vi "Supply_ComplianceCheck.vi"(8 "error in (no error)":errorcluster, 11 "KE2657A in":refnum<class "KE2657A.lvclass">) -> (0 "error out":errorcluster, 1 "Status string":string, 2 "Compliance exceeded?":bool, 3 "KE2657A out":refnum<class "KE2657A.lvclass">)   [LabVIEW 2018]
uses:
  KE2657A.lvclass
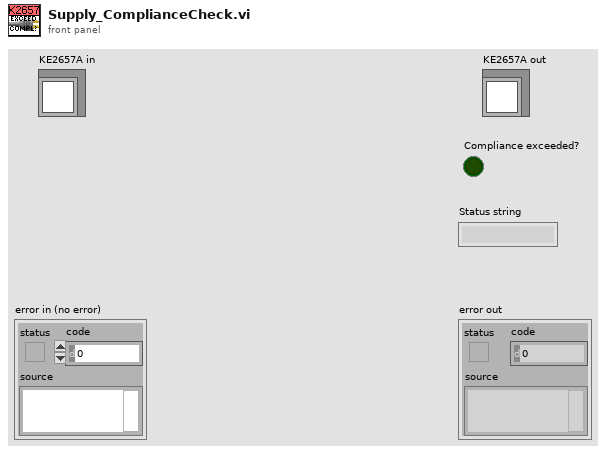
[diagram p1: front panel]
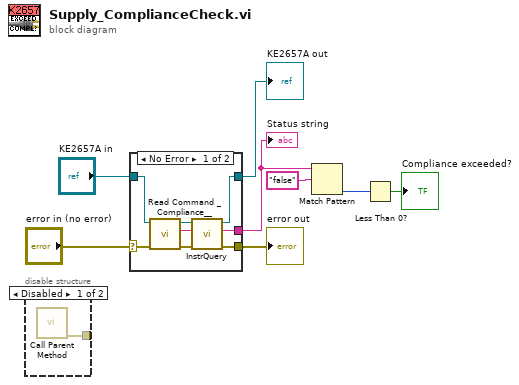
[diagram p0: block diagram]
diagram:
  n1 = disable-structure shown="Disabled" {
    disable-tunnel: [w9 _] -> _
    frame Disabled {
      n2 = call-parent "Call Parent Method"() -> ("error out"=w9:errorcluster)  [unwired: 8 in, 3 out]
    }
    frame Enabled {
    }
  }
  n3 = case shown="No Error" "error in (no error)" {
    selector: "error in (no error)" -> [w10 w18]
    tunnel: [w17 w18] -> w5
    tunnel: [w16 w19] -> w6
    tunnel: "KE2657A in" -> [w12 w19]
    tunnel: [w11 _] -> w4
    frame No Error {
      n4 = call-dynamic "Read Command _Compliance__.vi"("error in (no error)"=w10, "SupplyControl in"=w12) -> ("error out"=w15:errorcluster, "Command \"Compliance?\""=w14:string, "SupplyControl out"=w13:refnum<class "KE2657A.lvclass">)  [unwired: 7 in]
      n5 = call-dynamic "InstrQuery.vi"("error in (no error)"=w15, "Command string"=w14, "InstControl in"=w13) -> ("error out"=w17:errorcluster, "Instrument response"=w11:string, "InstControl out"=w16:refnum<class "KE2657A.lvclass">)  [unwired: 6 in]
    }
    frame Error {
    }
  }
  "KE2657A out" <- w6
  "error out" <- w5
  "Status string" <- w4
  n6 = Match Pattern(string=w4, regular expression="false") -> (offset past match=w2:i32)  [unwired: 1 in, 3 out]
  n7 = Less Than 0?(x=w2) -> (x < 0?=→"Compliance exceeded?":bool)
